vi "Add Publisher.vi"(8 "error in (no error)":errorcluster, 9 "Publication Type (TBD)":variant, 10 "Publisher Name":string, 11 "Topic in":refnum<class "Topic.lvclass">) -> (0 "error out":errorcluster, 3 "Topic out":refnum<class "Topic.lvclass">)   [LabVIEW 2015, in "Mediator.lvlib" / "Topic.lvclass"]
uses:
  Topic.lvclass
  Topic.lvclass/Topic.ctl
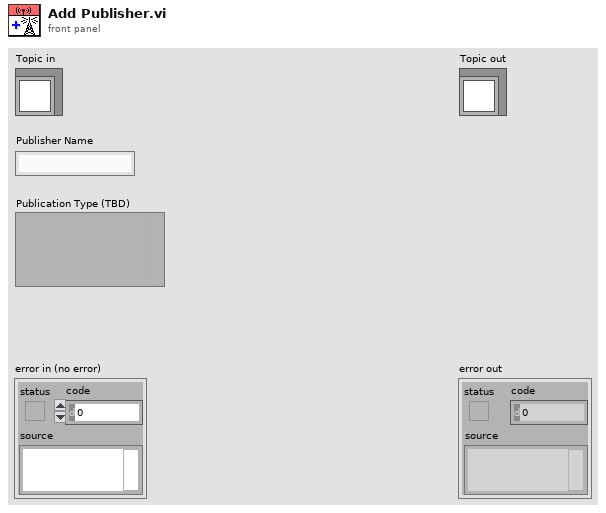
[diagram p1: front panel]
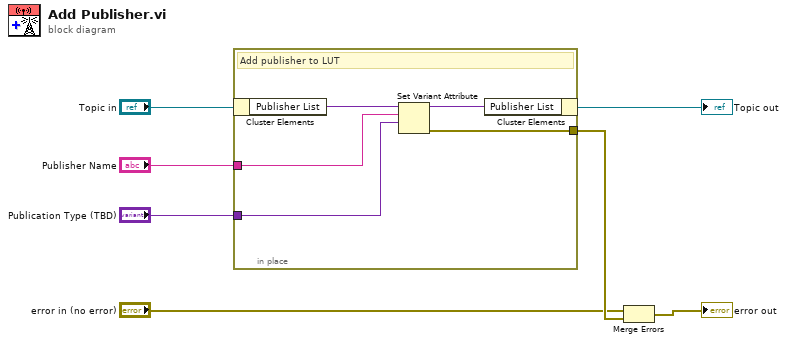
[diagram p0: block diagram]
diagram:
  n1 = in-place {
    in-place-border: [w10] -> w7
    in-place-border: "Publisher Name" -> [w9]
    in-place-border: "Publication Type (TBD)" -> [w8]
    # "Add publisher to LUT"
    n2 = in-place-cluster #1("Topic in") -> ("Publisher List"=w12:variant)
    n3 = Set Variant Attribute(Variant=w12, name=w9, value=w8) -> (Variant out=w11:variant, error out=w10:errorcluster)  [unwired: 1 in, 1 out]
    n4 = in-place-cluster #1("Publisher List"=w11) -> (→"Topic out":refnum<class "Topic.lvclass">)
  }
  n5 = Merge Errors("error in (no error)", w7) -> (→"error out":errorcluster)
